vi "PNG String 2 Picture.vi"(8 "error in (no error)":errorcluster, 10 "PNG Data as String":string, 11 "Picture In":picture) -> (0 "error out":errorcluster, 3 "Picture Out":picture)   [LabVIEW 2012]
doc: "Converts a string of raw PNG encoded data into a LabVIEW Picture."
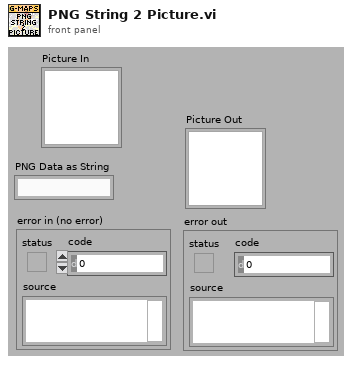
[diagram p1: front panel]
types:
  T1 = typedef "imagedata.ctl" = cluster{"image type":i32, "image depth":i32, "image":u8[], "mask":u8[], "colors":u32[], "Rectangle":cluster{"left":i16, "top":i16, "right":i16, "bottom":i16}}
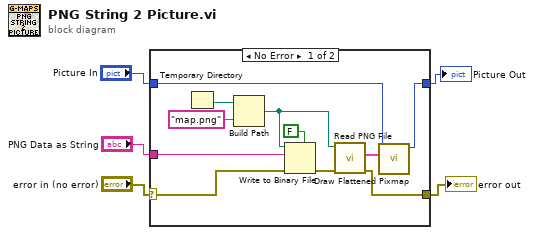
[diagram p0: block diagram]
diagram:
  n1 = case shown="No Error" "error in (no error)" {
    selector: "error in (no error)" -> [w7 w17]
    tunnel: [w16 w17] -> w2
    tunnel: [w15 w18] -> w1
    tunnel: "PNG Data as String" -> [w8 _]
    tunnel: "Picture In" -> [w6 w18]
    frame No Error {
      n2 = Temporary Directory() -> (w9:path)
      n3 = Build Path(base path=w9, name or relative path="map.png") -> (appended path=w11:path)
      n4 = Write to Binary File(file (use dialog)=w11, data=w8, error in=w7, 5:FALSE ("prepend array or string size? (T)")) -> (error out=w12:errorcluster)  [unwired: 2 in, 2 out]
      n5 = call <vilib>:"Read PNG File.vi"("error in (no error)"=w12, "path to PNG file"=w11) -> ("error out"=w16:errorcluster, "image data"=w14:T1)  [unwired: 7 in, 1 out]
      n6 = call <vilib>:"Draw Flattened Pixmap.vi"("image data"=w14, "picture"=w6) -> ("new picture"=w15:picture)  [unwired: 7 in]
    }
    frame Error {
    }
  }
  "error out" <- w2
  "Picture Out" <- w1
